vi "Setup UI.vi"(8 "error in (no error)":errorcluster, 10 "Set UI to input? (F)":bool, 11 "Power Meter in":refnum<class "Power Meter.lvclass">) -> (0 "error out":errorcluster, 3 "Power Meter out":refnum<class "Power Meter.lvclass">)   [LabVIEW 2015, in "Power Meter.lvclass"]
doc: "Setup UI constructs an object -- populates its member fields -- from a front panel the user can see. The VI should be as simple as possible so that a UI loop can poll it continuously for updates. \n\nThe VI is designed to be used as a subPanel within another VI. Wire true to \"Set UI to input\" only on the first call, just after inserting this VI into a subPanel, to populate its controls with the class's current values.\n\nSetup UI is distinct from the class constructor. Class constructors are not polymorphic, yet configure dialogs need to configure objects without knowing their type -- and polymorphism is the necessary solution. Thus, Setup UI is a polymorphic class constructor. This continously polled \"Setup UI\" concept is a kludge: a better idea would be an XControl, but those require a steeper learning curve."
uses:
  Power Meter.lvclass
  Newport 1830-C/Public/Filters.ctl
  Power Meter.lvclass/Power Meter.ctl
  Utility Classes/Readable/Readable.lvclass
  Newport 1830-C/Newport 1830-C.lvlib
panel:
  in  "Filter":T1=1 items=["Orange"=1, "Green"=2, "Yellow"=3]
  in  "Set":bool
  in  "ATTN":u32(ring) items=["Off", "On"]
  in  "Range":u32(ring) items=["Auto", "Lowest", "2", "3", "4", "5", "6", "7", "Highest"]
  in  "AVG":u32(ring)=2 items=["Slow"=1, "Medium"=2, "Fast"=3]
  in  "Wavelength":dbl[unit]=7.8e-07
  # "Power Meter Setup"
  # "Initializes to current\nrange only: never\nAuto-Ranging"
  # "Slow-> Ave of 16\nMed-> Ave of 4\nFast-> No Ave"
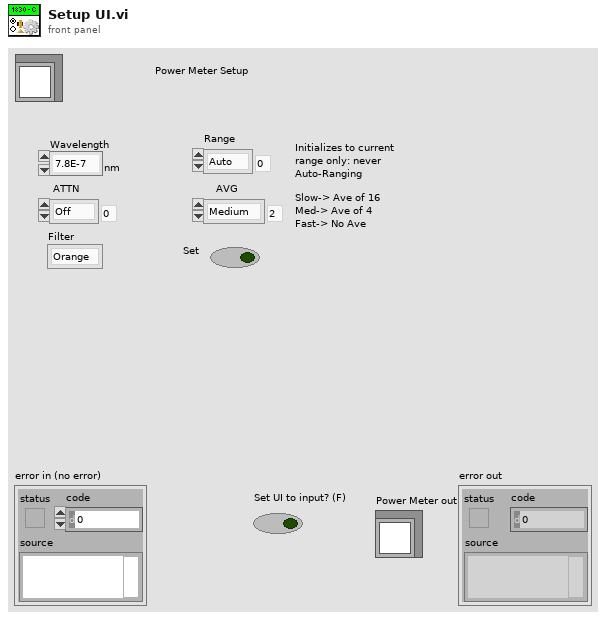
[diagram p1: front panel]
types:
  T1 = typedef "Filters.ctl" = u16
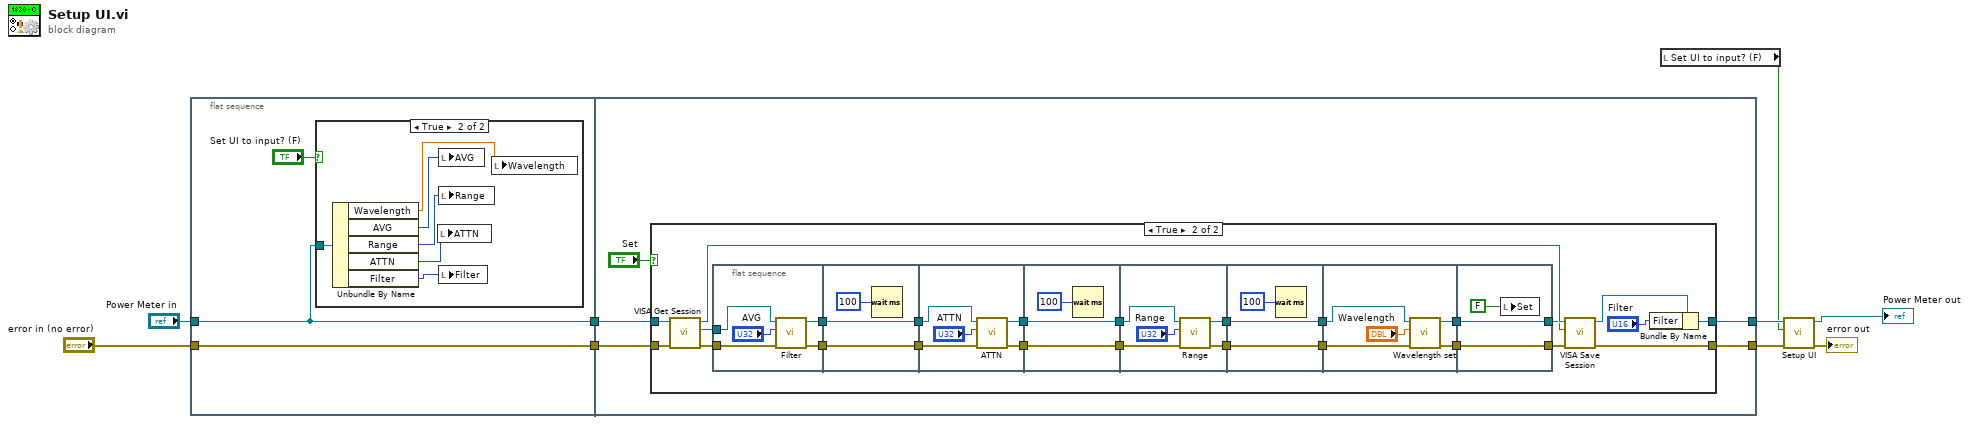
[diagram p0: block diagram]
diagram:
  n1 = flat-sequence {
    tunnel: "Power Meter in" -> [w11]
    tunnel: [w11] -> w7
    tunnel: "error in (no error)" -> [w10]
    tunnel: [w10] -> w5
    tunnel: w7 -> [w23]
    tunnel: w5 -> [w22]
    tunnel: [w20] -> w4
    tunnel: [w19] -> w3
    frame #0 {
      n2 = case shown="True" "Set UI to input? (F)" {
        tunnel: w11 -> [_ w18]
        frame False {
        }
        frame True {
          n3 = Unbundle By Name(w18) -> ("Wavelength"=w17:dbl[unit], "AVG"=w16:u16, "Range"=w15:u16, "ATTN"=w14:u16, "Filter"=w13:T1)
          n4 = local write "ATTN"(w14) -> ()
          n5 = local write "AVG"(w16) -> ()
          n6 = local write "Range"(w15) -> ()
          n7 = local write "Filter"(w13) -> ()
          n8 = local write "Wavelength"(w17) -> ()
        }
      }
    }
    frame #1 {
      n9 = case shown="True" "Set" {
        tunnel: w23 -> [w25 w50]
        tunnel: w22 -> [w24 w49]
        tunnel: [w25 w26] -> w20
        tunnel: [w24 w29] -> w19
        frame False {
        }
        frame True {
          n10 = call-dynamic "VISA Get Session.vi"("error in (no error)"=w49, "Instrument.lvclass in"=w50) -> ("error out"=w47:errorcluster, "VISA Resource Name"=w48:refnum<visa-resource-name>, "Instrument.lvclass out"=w34:refnum<class "Power Meter.lvclass">)  [unwired: 6 in, 1 out]
          n11 = flat-sequence {
            tunnel: w48 -> [w54]
            tunnel: w47 -> [w53]
            tunnel: [w52] -> w45
            tunnel: [w51] -> w43
            tunnel: [w57] -> w46
            tunnel: w45 -> [w57]
            tunnel: [w56] -> w44
            tunnel: w43 -> [w56]
            tunnel: w46 -> [w63]
            tunnel: w44 -> [w62]
            tunnel: [w60] -> w41
            tunnel: [w59] -> w39
            tunnel: [w65] -> w42
            tunnel: w41 -> [w65]
            tunnel: [w64] -> w40
            tunnel: w39 -> [w64]
            tunnel: w42 -> [w71]
            tunnel: w40 -> [w70]
            tunnel: [w68] -> w37
            tunnel: [w67] -> w35
            tunnel: [w73] -> w38
            tunnel: w37 -> [w73]
            tunnel: [w72] -> w36
            tunnel: w35 -> [w72]
            tunnel: w38 -> [w78]
            tunnel: w36 -> [w77]
            tunnel: [w76] -> w33
            tunnel: [w75] -> w31
            tunnel: w33 -> [w81]
            tunnel: [w81] -> w32
            tunnel: [w80] -> w30
            tunnel: w31 -> [w80]
            frame #0 {
              n12 = call "Filter.vi"("error in (no error)"=w53, "Filter"="AVG", "VISA resource name"=w54) -> ("error out"=w52:errorcluster, "VISA resource name out"=w51:refnum<visa-resource-name>)  [unwired: 7 in]
            }
            frame #1 {
              n13 = Wait (ms)(milliseconds to wait=u32 100) -> ()  [unwired: 1 out]
            }
            frame #2 {
              n14 = call "ATTN.vi"("error in (no error)"=w63, "Attn"="ATTN", "VISA resource name"=w62) -> ("error out"=w59:errorcluster, "VISA resource name out"=w60:refnum<visa-resource-name>)  [unwired: 7 in]
            }
            frame #3 {
              n15 = Wait (ms)(milliseconds to wait=u32 100) -> ()  [unwired: 1 out]
            }
            frame #4 {
              n16 = call "Range.vi"("error in (no error)"=w70, "Range"="Range", "VISA resource name"=w71) -> ("error out"=w67:errorcluster, "VISA resource name out"=w68:refnum<visa-resource-name>)  [unwired: 7 in]
            }
            frame #5 {
              n17 = Wait (ms)(milliseconds to wait=u32 100) -> ()  [unwired: 1 out]
            }
            frame #6 {
              n18 = call "Wavelength set.vi"("error in (no error)"=w77, "Wavelength (nnnn)"="Wavelength", "VISA resource name"=w78) -> ("error out"=w75:errorcluster, "VISA resource name out"=w76:refnum<visa-resource-name>)  [unwired: 7 in]
            }
            frame #7 {
              n19 = local write "Set"(FALSE ("Set")) -> ()
            }
          }
          n20 = call-dynamic "VISA Save Session.vi"("error in (no error)"=w30, "VISA Resource Name"=w32, "Instrument.lvclass in"=w34) -> ("error out"=w29:errorcluster, "Instrument.lvclass out"=w28:refnum<class "Power Meter.lvclass">)  [unwired: 7 in]
          n21 = Bundle By Name(cluster=w28, "Filter"="Filter") -> (w26:refnum<class "Power Meter.lvclass">)
        }
      }
    }
  }
  n22 = local read "Set UI to input? (F)"() -> (w2:bool)
  n23 = call-parent "Setup UI.vi"("error in (no error)"=w3, "Set UI to input? (F)"=w2, "Instrument in"=w4) -> ("error out"=→"error out":errorcluster, "Instrument out"=→"Power Meter out":refnum<class "Power Meter.lvclass">)  [unwired: 7 in]
